vi "String Remove Between.vi"(8 "End String":string, 9 "Start String":string, 10 "Input String":string) -> (1 "Resultant String":string)   [LabVIEW 2011]
doc: "Removes the substring between two strings and returns the original string without the substring in between.\n\n<b>Input String</b> - String to search.\n\n<b>Start String</b> - String to find that designates the start of the string to find.\n\n<b>End String</b> - String to find that designates the end of the string to find.\n\nExample:\n<b>Input String</b>This String has a comment /test/in it.\n<b>Start String</b>/\n<b>End String</b>/\n<b>Resultant String</b> This String has a comment in it.\n\n\nVersion 1.0 - 10/20/2009\n\nPhaeron, Inc.\nwww.phaeron.com\ninfo@phaeron.com"
panel:
  out "offset past match":i32
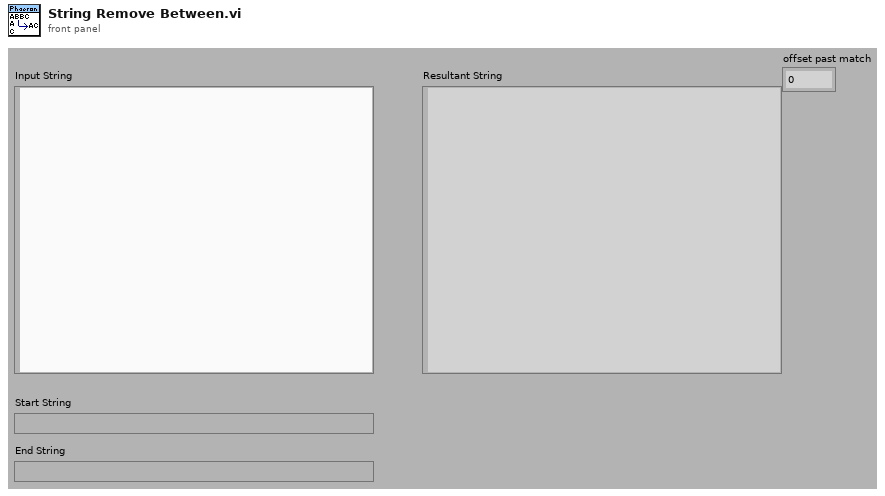
[diagram p1: front panel]
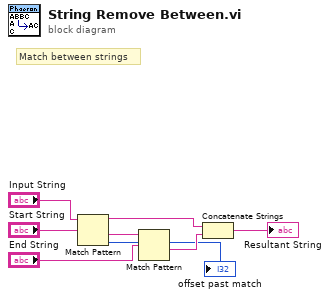
[diagram p0: block diagram]
diagram:
  # "Match between strings"
  n1 = Match Pattern(string="Input String", regular expression="Start String") -> (before substring=w4:string, after substring=w5:string, offset past match=→"offset past match":i32)  [unwired: 1 in, 1 out]
  n2 = Match Pattern(string=w5, regular expression="End String") -> (after substring=w3:string)  [unwired: 1 in, 3 out]
  n3 = Concatenate Strings(w4, w3) -> (→"Resultant String":string)
